vi "Build Result File Path.vi"(0 "Charact Result Accessor in":refnum<class "Charact Result Accessor.lvclass">, 5 "Output Directory":path, 7 "Port 1":string, 9 "Port 2":string, 11 "error in (no error)":errorcluster) -> (4 "Charact Result Accessor out":refnum<class "Charact Result Accessor.lvclass">, 6 "Result File Path":path, 15 "error out":errorcluster)   [LabVIEW 2023, in "RFFixtureCharact.RFPM.lvlib" / "Charact Result Accessor.lvclass"]
uses:
  Charact Result Accessor.lvclass
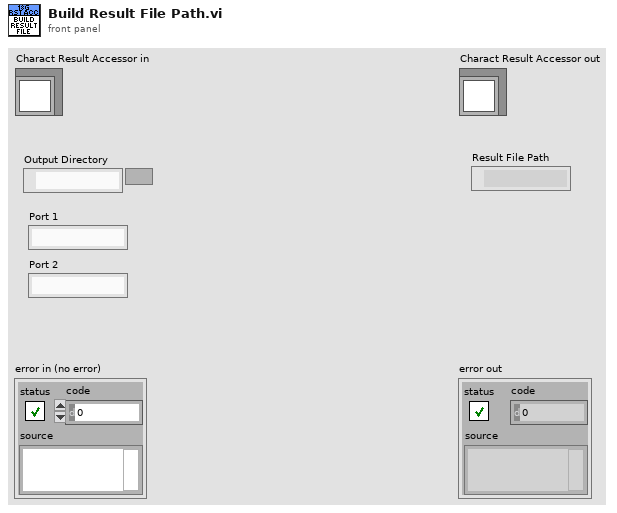
[diagram p1: front panel]
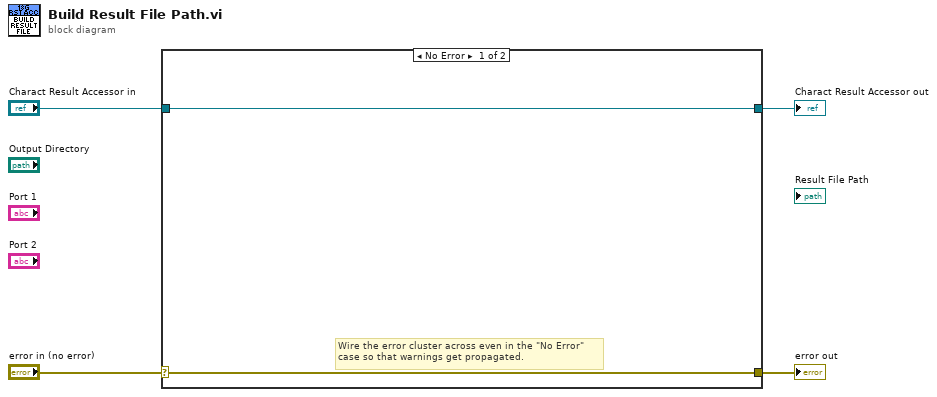
[diagram p0: block diagram]
diagram:
  n1 = case shown="No Error" "error in (no error)" {
    selector: "error in (no error)" -> [w5 w8]
    tunnel: [w5 w8] -> w3
    tunnel: [w6 w7] -> w1
    tunnel: "Charact Result Accessor in" -> [w6 w7]
    frame No Error {
      # "Wire the error cluster across even in the \"No Error\"\ncase so that warnings get propagated."
    }
    frame Error {
    }
  }
  "error out" <- w3
  "Charact Result Accessor out" <- w1
